vi "Read HW Config Class.vi"(8 "error in (no error)":errorcluster, 11 "Hardware in":refnum<class "Hardware.lvclass">) -> (0 "error out":errorcluster, 2 "Hardware.lvlib:HW Configuration.lvclass":refnum<class "HW Configuration.lvclass">, 3 "Hardware out":refnum<class "Hardware.lvclass">)   [LabVIEW 2026, in "Hardware.lvlib" / "Hardware.lvclass"]
uses:
  Hardware.lvclass
  HW Config/HW Configuration.lvclass
  Hardware.lvclass/Hardware.ctl
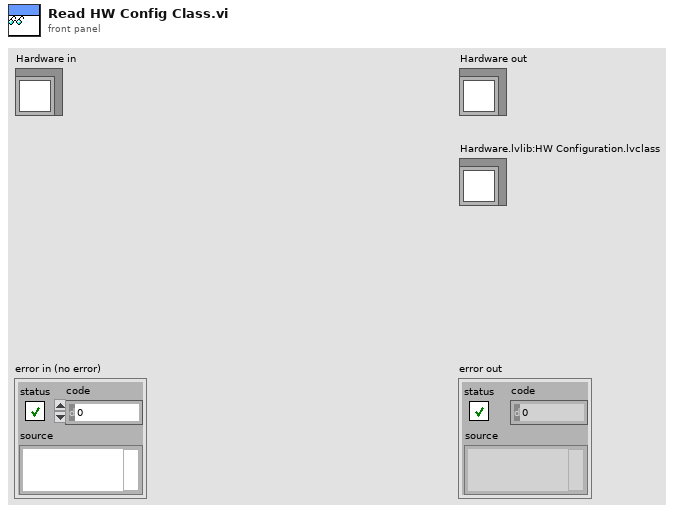
[diagram p1: front panel]
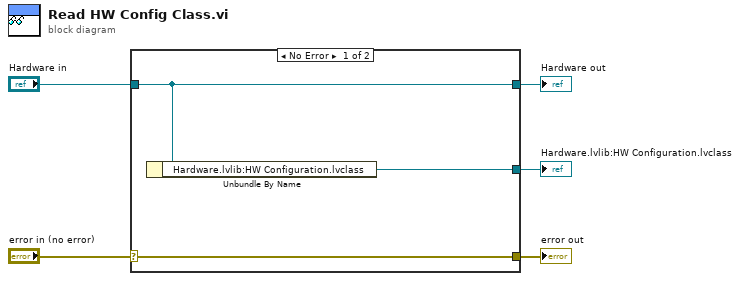
[diagram p0: block diagram]
diagram:
  n1 = case shown="No Error" "error in (no error)" {
    selector: "error in (no error)" -> [w8 w9]
    tunnel: [w8 w9] -> w4
    tunnel: [w7 w10] -> w2
    tunnel: "Hardware in" -> [w7 w10]
    tunnel: [w6 _] -> w1
    frame No Error {
      n2 = Unbundle By Name(w7) -> ("Hardware.lvlib:HW Configuration.lvclass"=w6:refnum<class "HW Configuration.lvclass">)
    }
    frame Error {
    }
  }
  "error out" <- w4
  "Hardware out" <- w2
  "Hardware.lvlib:HW Configuration.lvclass" <- w1
